vi "Close.vi"(8 "error in":errorcluster, 11 "HH802U in":refnum<class "HH802U.lvclass">) -> (0 "error out":errorcluster, 3 "HH802U out":refnum<class "HH802U.lvclass">)   [LabVIEW 2015, in "HH802U.lvclass"]
uses:
  HH802U.lvclass
  HH802U.lvclass/HH802U.ctl
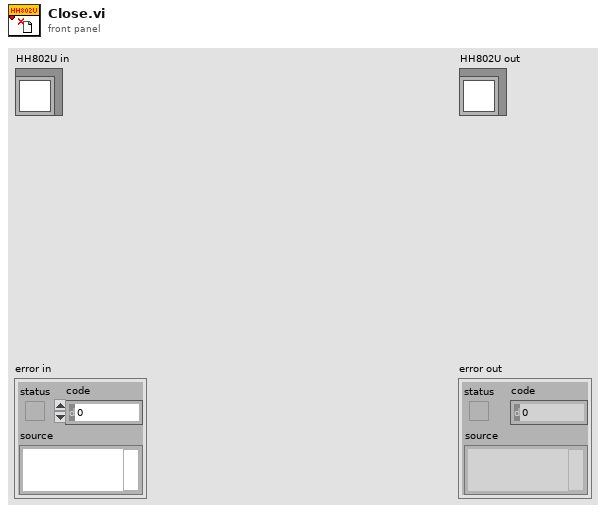
[diagram p1: front panel]
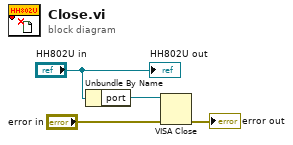
[diagram p0: block diagram]
diagram:
  n1 = Unbundle By Name("HH802U in") -> ("port"=w3:refnum<visa-resource-name>)
  n2 = VISA Close(VISA resource name=w3, error in (no error)="error in") -> (error out=→"error out":errorcluster)
  "HH802U out" <- "HH802U in"
